vi "Set Chronometer.vi"(8 "error in":errorcluster, 11 "Report in":refnum<class "Report.lvclass">) -> (0 "error out":errorcluster, 3 "Report out":refnum<class "Report.lvclass">)   [LabVIEW 2019]
uses:
  PPL/Chronometer.lvlibp/Chronometer.lvclass
  Report.lvclass
  C:/Users/rdexter/Documents/Development/Drivers/PPL/Instruments.lvlibp/Instruments.lvclass
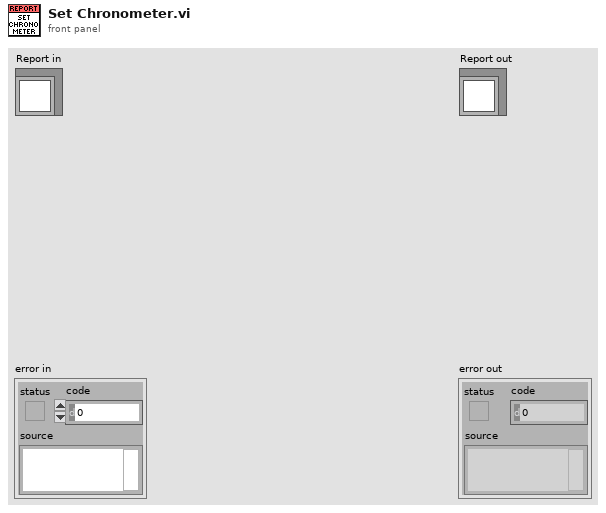
[diagram p1: front panel]
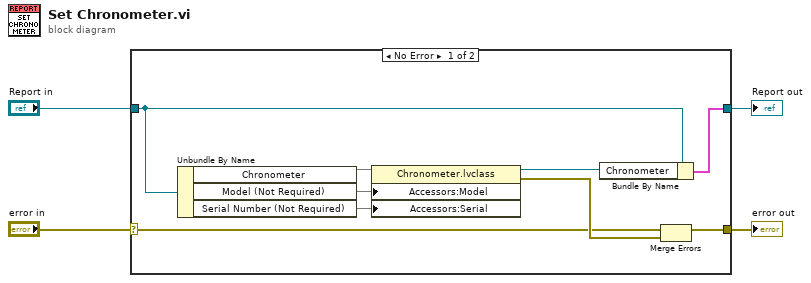
[diagram p0: block diagram]
diagram:
  n1 = case shown="No Error" "error in" {
    selector: "error in" -> [w5 w15]
    tunnel: [w6 w15] -> w3
    tunnel: [w12 w14] -> w1
    tunnel: "Report in" -> [w13 w14]
    frame No Error {
      n2 = Unbundle By Name(w13) -> ("Chronometer"=w11, "Model (Not Required)"=w9, "Serial Number (Not Required)"=w8)
      n3 = property class="Chronometer.lvclass"(reference=w11, "Accessors:Model"=w9, "Accessors:Serial"=w8) -> (reference out=w10:refnum<class "Chronometer.lvclass">, error out=w7:errorcluster)  [unwired: 1 in]
      n4 = Bundle By Name(cluster=w13, "Chronometer"=w10) -> (w12:cluster{})
      n5 = Merge Errors(w5, w7) -> (w6:errorcluster)
    }
    frame Error {
    }
  }
  "error out" <- w3
  "Report out" <- w1
